vi "Config Test.vi"() -> ()   [LabVIEW 2015, in "ResultProcessor Tests.lvlib"]
uses:
  ResultProcessor Tests.lvlib
  Config/ResultProcessor Config.lvclass
  Report/On-The-Fly/Config/OnTheFlyReport Config.lvclass
  Report Formatters/csv/Config/csv-formatter Config.lvclass
panel:
  out "x = y?":bool
  out "ResultProcessor Config out":refnum<class "ResultProcessor Config.lvclass">
  out "data":string
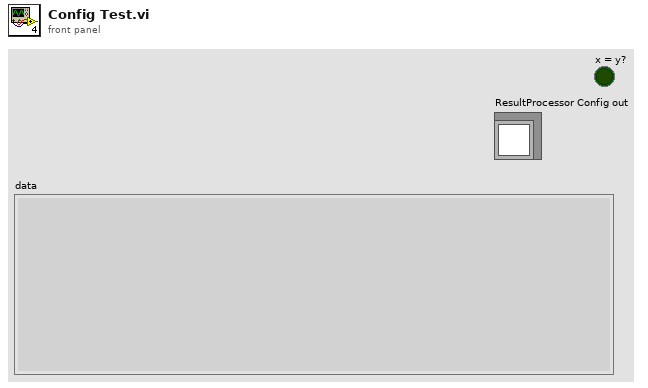
[diagram p1: front panel]
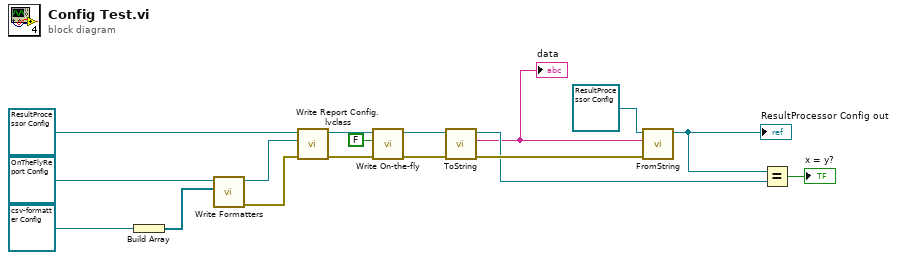
[diagram p0: block diagram]
diagram:
  n1 = Build Array(refnum<class "csv-formatter Config.lvclass"> refnum ("csv-formatter Config.lvclass")) -> (w8:refnum<class "csv-formatter Config.lvclass">[])
  n2 = call-dynamic "Write Formatters.vi"("Formatters"=w8, "OnTheFlyReport Config in"=refnum<class "OnTheFlyReport Config.lvclass"> refnum ("OnTheFlyReport Config.lvclass")) -> ("error out"=w7:errorcluster, "OnTheFlyReport Config out"=w10:refnum<class "OnTheFlyReport Config.lvclass">)  [unwired: 8 in]
  n3 = call-dynamic "Write Report Config.lvclass.vi"("error in (no error)"=w7, "Report Config.lvclass"=w10, "ResultProcessor Config in"=refnum<class "ResultProcessor Config.lvclass"> refnum) -> ("error out"=w4:errorcluster, "ResultProcessor Config out"=w11:refnum<class "ResultProcessor Config.lvclass">)  [unwired: 7 in]
  n4 = call-dynamic "Write On-the-fly.vi"("error in (no error)"=w4, "On-the-fly?"=FALSE, "ResultProcessor Config in"=w11) -> ("error out"=w3:errorcluster, "ResultProcessor Config out"=w5:refnum<class "ResultProcessor Config.lvclass">)  [unwired: 7 in]
  n5 = call-dynamic "ToString.vi"("error in (no error)"=w3, "ResultProcessor Config in"=w5) -> ("error out"=w17:errorcluster, "data"=w13:string, "ResultProcessor Config out"=w15:refnum<class "ResultProcessor Config.lvclass">)  [unwired: 7 in]
  "data" <- w13
  n6 = call-dynamic "FromString.vi"("error in (no error)"=w17, "data"=w13, "ResultProcessor Config in"=refnum<class "ResultProcessor Config.lvclass"> refnum) -> ("ResultProcessor Config out"=w6:refnum<class "ResultProcessor Config.lvclass">)  [unwired: 7 in, 1 out]
  "ResultProcessor Config out" <- w6
  n7 = Equal?(x=w6, y=w15) -> (x = y?=→"x = y?":bool)
